vi "RTL-SDR Init App Defaults.vi"(8 "error in (no error)":errorcluster, 11 "RTL-SDR Device In":u64) -> (0 "error out":errorcluster, 3 "RTL-SDR Device Out":u64)   [LabVIEW 2016]
doc: "Initialise RTL-SDR to default values for this application."
uses:
  <vilib>/rtlsdr/rtlsdr.lvlib
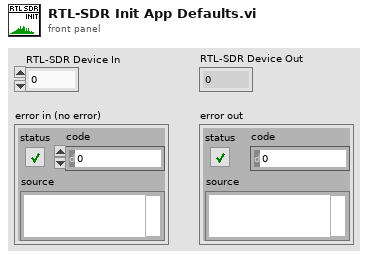
[diagram p1: front panel]
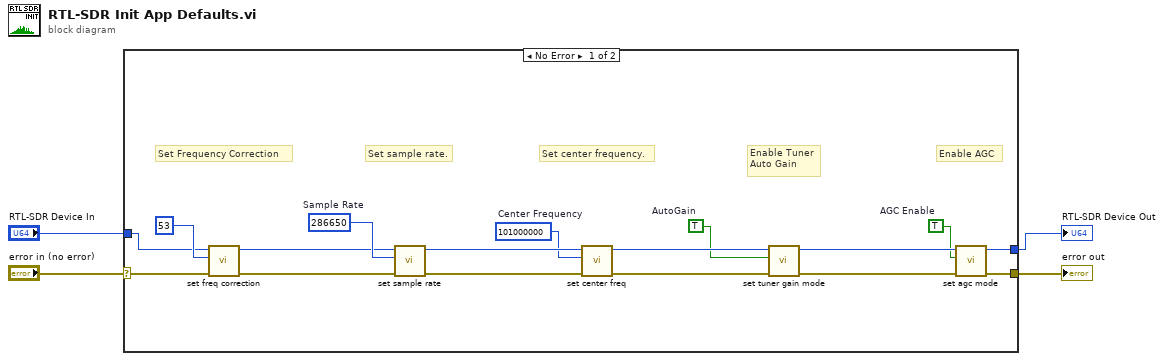
[diagram p0: block diagram]
diagram:
  n1 = case shown="No Error" "error in (no error)" {
    selector: "error in (no error)" -> [w5 w22]
    tunnel: [w20 w23] -> w4
    tunnel: [w19 w22] -> w3
    tunnel: "RTL-SDR Device In" -> [w6 w23]
    frame No Error {
      w9 = u32 101000000  # Center Frequency
      w8 = TRUE  # AutoGain
      w7 = TRUE  # AGC Enable
      w21 = u32 286650  # Sample Rate
      # "Set Frequency Correction"
      # "Enable Tuner\nAuto Gain"
      # "Enable AGC"
      # "Set center frequency."
      # "Set sample rate."
      n2 = call <vilib>:"set freq correction.vi"("error in (no error)"=w5, "Frequency Correction (ppm)"=53, "DeviceRefnum"=w6) -> ("error out"=w16:errorcluster, "DeviceRefnum Out"=w18:u64)  [unwired: 6 in, 1 out]
      n3 = call <vilib>:"set sample rate.vi"("error in (no error)"=w16, "Sample Rate"=w21, "DeviceRefnum"=w18) -> ("error out"=w10:errorcluster, "DeviceRefnum Out"=w11:u64)  [unwired: 6 in, 1 out]
      n4 = call <vilib>:"set center freq.vi"("error in (no error)"=w10, "Center Frequency"=w9, "DeviceRefnum"=w11) -> ("error out"=w15:errorcluster, "DeviceRefnum Out"=w12:u64)  [unwired: 6 in, 1 out]
      n5 = call <vilib>:"set tuner gain mode.vi"("error in (no error)"=w15, "AutoGain"=w8, "DeviceRefnum"=w12) -> ("error out"=w14:errorcluster, "DeviceRefnum Out"=w13:u64)  [unwired: 6 in, 1 out]
      n6 = call <vilib>:"set agc mode.vi"("error in (no error)"=w14, "AGC Enable"=w7, "DeviceRefnum"=w13) -> ("error out"=w19:errorcluster, "DeviceRefnum Out"=w20:u64)  [unwired: 6 in, 1 out]
    }
    frame Error {
    }
  }
  "RTL-SDR Device Out" <- w4
  "error out" <- w3
